vi "GetProcessFullName.vi"(8 "error in":errorcluster, 11 "OperationRun in":refnum<class "OperationRun.lvclass">) -> (0 "error out":errorcluster, 2 "ProcessFullName":string, 3 "OperationRun out":refnum<class "OperationRun.lvclass">)   [LabVIEW 2021, in "ProligentXMLGenerator.lvlib" / "OperationRun.lvclass"]
doc: "Defines the input format for a Process FullName\n\"[Root Process/][[Path/]...]Name\"\nEach path strings and the name are limited to 64 characters and the total string provided is limited to 1900 characters\n\nWARNING:\n\nSince the '/' character is the hierarchy delimiter, if a path string contains a '/' character it will be interpreted as\na new hierarchy. It is therefore suggested to replace '/' by '-' in all your path components to keep the expected hierarchy.\nFor example, if you have a sequence named 'PASS/FAIL' and you don't substitude '/' by '-', the 'PASS' would be interpreted\nas a sequence category while 'FAIL' would be the name of a sequence. If you do the suggested substitution, the name of\nthe sequence would be interpreted as 'PASS-FAIL' without any category."
uses:
  OperationRun.lvclass
  OperationRun.lvclass/OperationRun.ctl
  Base/ProcessFullName/ProcessFullName.lvclass
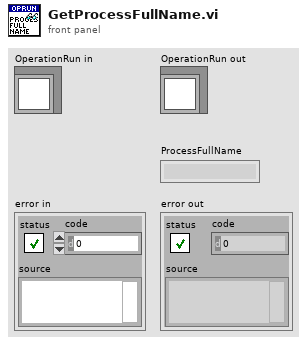
[diagram p1: front panel]
types:
  T1 = typedef "ProligentXMLGenerator.lvlib/OperationRun.lvclass/Data.ctl" = cluster{"Name":string, "Characteristics":refnum<class "Characteristic.lvclass">[], "Documents":refnum<class "Document.lvclass">[], "SequenceRuns":refnum<class "SequenceRun.lvclass">[], "FailureReferences":refnum<class "FailureReference.lvclass">[], "SequenceRunReferences":refnum<class "SequenceRunReference.lvclass">[], "CustomData":refnum<class "CustomData.lvclass">, "OperationRunId":refnum<class "Guid.lvclass">, "ProcessFullName":refnum<class "ProcessFullName.lvclass">, "ProcessVersion":refnum<class "NonEmptyString_64.lvclass">, "OperationName":refnum<class "NonEmptyString_65.lvclass">, "StationFullName":refnum<class "FullName.lvclass">, "User":refnum<class "NonEmptyString_255.lvclass">, "CallingOperationRunId":refnum<class "Guid.lvclass">, "OperationStatus":refnum<class "ExecutionStatus.lvclass">, "OperationRunStartTime":refnum<class "DateTime.lvclass">, "OperationRunEndTime":refnum<class "DateTime.lvclass">, "TimeZoneInfoId":string}
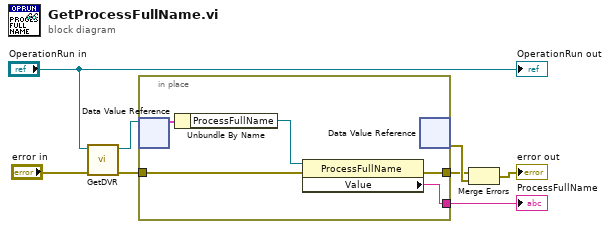
[diagram p0: block diagram]
diagram:
  n1 = call "GetDVR.vi"("error in"="error in", "OperationRun"="OperationRun in") -> ("error out"=w2:errorcluster, "DVRReference"=w7:refnum<data-value>)  [unwired: 8 in]
  n2 = in-place "In Place Element Structure" {
    in-place-border: [w10] -> w6
    in-place-border: w2 -> [w11]
    in-place-border: [w9] -> w1
    n3 = in-place-dvr #1(w7) -> (w13:T1)  [unwired: 1 out]
    n4 = Unbundle By Name(w13) -> ("ProcessFullName"=w12:refnum<class "ProcessFullName.lvclass">)
    n5 = property on="Property Node" class="ProcessFullName"(reference=w12, error in=w11) -> (error out=w9:errorcluster, "Value"=w10:string)  [unwired: 1 out]
    n6 = in-place-dvr #1() -> (w8:errorcluster)  [unwired: 1 in, 1 out]
  }
  "ProcessFullName" <- w6
  n7 = Merge Errors(w1, w8) -> (→"error out":errorcluster)
  "OperationRun out" <- "OperationRun in"
